vi "getUsage.vi"(6 "timeout (10000)":i32=10000, 8 "error in (no error)":errorcluster, 11 "Parameters":T2) -> (0 "error out":errorcluster, 3 "Response":T1, 4 "error data":string[](array[string]))   [LabVIEW 2017, in "Random JSON API.lvlib"]
uses:
  Random JSON API.lvlib
  Type Defs/getUsageRequest.ctl
  Type Defs/getUsageResponse.ctl
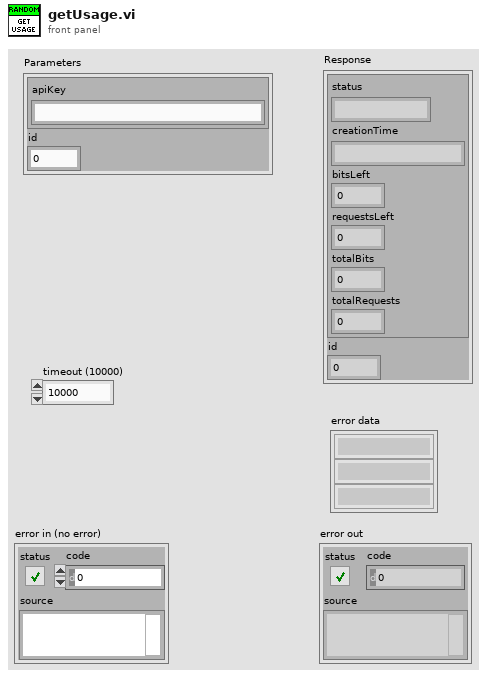
[diagram p1: front panel]
types:
  T1 = typedef "Random JSON API.lvlib/getUsageResponse.ctl" = cluster{"result":cluster{"status":string, "creationTime":string, "bitsLeft":i32, "requestsLeft":i32, "totalBits":i32, "totalRequests":i32}, "id":dbl}
  T2 = typedef "Random JSON API.lvlib/getUsageRequest.ctl" = cluster{"params":cluster{"apiKey":string}, "id":dbl}
  T3 = cluster{"jsonrpc":string, "method":string, "params":cluster{"apiKey":string}, "id":dbl}
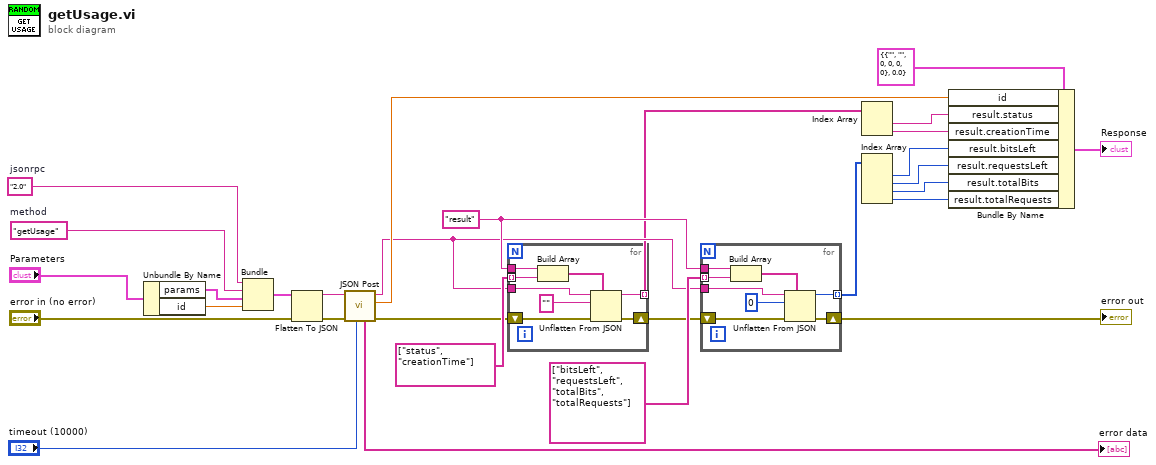
[diagram p0: block diagram]
diagram:
  w17 = "result"
  w24 = "2.0"  # jsonrpc
  w23 = "getUsage"  # method
  n1 = Unbundle By Name("Parameters") -> ("params"=w22:cluster{"apiKey":string}, "id"=w21:dbl)
  n2 = Bundle("jsonrpc"=w24, "method"=w23, "params"=w22, "id"=w21) -> (w20:T3)  [unwired: 1 in]
  n3 = Flatten To JSON(anything=w20, error in (no error)="error in (no error)") -> (JSON string=w27:string, 11:w26:errorcluster)  [unwired: 1 in]
  n4 = call "JSON Post.vi"("timeout (10000)"="timeout (10000)", "error in (no error)"=w26, "Request JSON String"=w27) -> ("error out"=w14:errorcluster, "id"=w19:dbl, "Response JSON String"=w15:string, "error data"=→"error data":string[])  [unwired: 5 in]
  n5 = for {
    shift-right: [w36] -> w13
    shift-left: w14 -> [w37]
    tunnel: [w35] -> w11 mode=indexing
    tunnel: w17 -> [w34]
    tunnel: string[] ["status", "creationTime"] -> [w32] mode=indexing
    tunnel: w15 -> [w31]
    n6 = Build Array(w34, w32) -> (w33:string[])
    n7 = Unflatten From JSON(path=w33, JSON string=w31, type and defaults="", error in (no error)=w37) -> (value=w35:string, error out=w36:errorcluster)  [unwired: 3 in]
  }
  n8 = for {
    shift-right: [w44] -> w12
    shift-left: w13 -> [w45]
    tunnel: [w42] -> w8 mode=indexing
    tunnel: w17 -> [w41]
    tunnel: string[] ["bitsLeft", "requestsLeft", "totalBits", "totalRequests"] -> [w39] mode=indexing
    tunnel: w15 -> [w38]
    n9 = Build Array(w41, w39) -> (w40:string[])
    n10 = Unflatten From JSON(path=w40, JSON string=w38, type and defaults=0, error in (no error)=w45) -> (value=w42:i32, error out=w44:errorcluster)  [unwired: 3 in]
  }
  "error out" <- w12
  n11 = Index Array(array=w11) -> (element #1=w10:string, element #2=w9:string)  [unwired: 2 in]
  n12 = Index Array(array=w8) -> (element #1=w7:i32, element #2=w4:i32, element #3=w5:i32, element #4=w6:i32)  [unwired: 4 in]
  n13 = Bundle By Name(cluster=T1 {"result"={"status"="", "creationTime"="", "bitsLeft"=0, "requestsLeft"=0, "totalBits"=0, "totalRequests"=0}, "id"=0.0} ("Response"), "id"=w19, "result.status"=w10, "result.creationTime"=w9, "result.bitsLeft"=w7, "result.requestsLeft"=w4, "result.totalBits"=w5, "result.totalRequests"=w6) -> (→"Response":T1)
